vi "10 DAQ Config (PFI0) (2017).vi"(2 "Error In":errorcluster, 3 "rate":dbl=6000.0, 4 "number of samples":i32=240) -> (0 "Error Out":errorcluster, 1 "task out":refnum<k21>)   [LabVIEW 2017]
uses:
  <vilib>/DAQmx/create/channels.llb/DAQmx Create Channel (TEDS-AI-Voltage-Basic).vi
  <vilib>/DAQmx/create/channels.llb/DAQmx Create Channel (AI-Voltage-Basic).vi
  <vilib>/DAQmx/configure/timing.llb/DAQmx Timing (Sample Clock).vi
  <vilib>/DAQmx/configure/trigger.llb/DAQmx Trigger.vi
  <vilib>/DAQmx/configure/trigger.llb/DAQmx Start Trigger (Digital Edge).vi
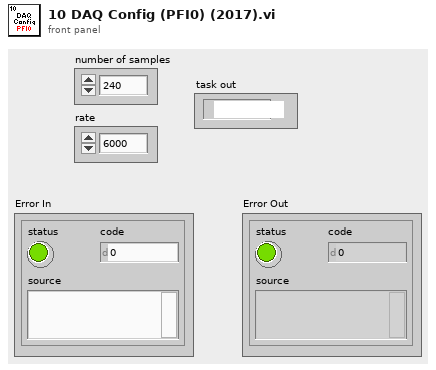
[diagram p1: front panel]
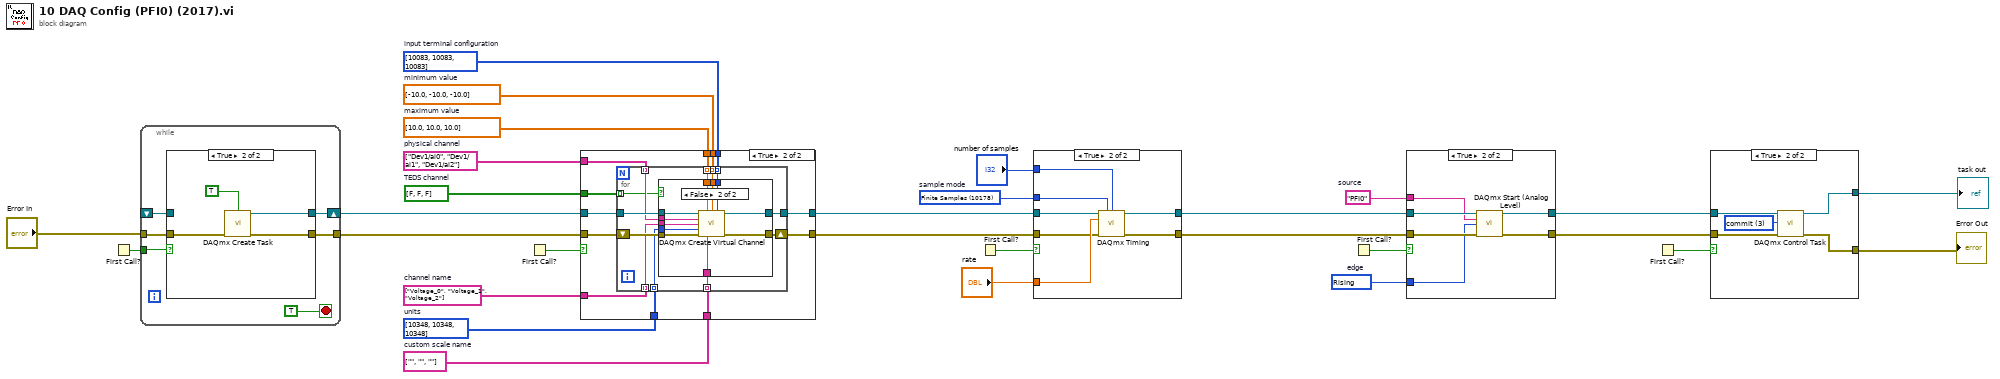
[diagram p0: block diagram]
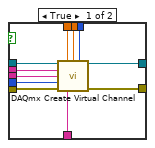
[diagram p6: hidden frame]
diagram:
  w26 = 10280 items=["Rising"=10280, "Falling"=10171]  # edge
  w25 = "PFI0"  # source
  w21 = 10178 items=["Finite Samples"=10178, "Continuous Samples"=10123, "Hardware Timed Single Point"=12522]  # sample mode
  w15 = bool[] [FALSE, FALSE, FALSE]  # TEDS channel
  w14 = string[] ["", "", ""]  # custom scale name
  w13 = i32[] [10348, 10348, 10348] items=["Volts"=10348, "From TEDS"=12516, "From Custom Scale"=10065]  # units
  w12 = string[] ["Voltage_0", "Voltage_1", "Voltage_2"]  # channel name
  w11 = string[] ["Dev1/ai0", "Dev1/ai1", "Dev1/ai2"]  # physical channel
  w10 = dbl[] [10.0, 10.0, 10.0]  # maximum value
  w9 = dbl[] [-10.0, -10.0, -10.0]  # minimum value
  w8 = i32[] [10083, 10083, 10083] items=["default"=-1, "RSE"=10083, "NRSE"=10078, "Differential"=10106, "Pseudodifferential"=12529]  # input terminal configuration
  n1 = First Call?() -> (First Call?: T/F=w3:bool)
  n2 = while {
    shift-right: [w34] -> w6
    shift-left: _ -> [w33]
    tunnel: w3 -> [w35]
    tunnel: [w32] -> w4
    tunnel: "Error In" -> [w31]
    stop <- TRUE stop-if-true
    n3 = case shown="True" w35 {
      tunnel: [w37 w41] -> w34
      tunnel: w33 -> [w37 _]
      tunnel: [w36 w40] -> w32
      tunnel: w31 -> [w36 w38]
      frame False {
      }
      frame True {
        n4 = call <vilib>:"DAQmx Create Task.vi"("auto cleanup"=TRUE, "error in"=w38) -> ("task out"=w41:refnum<k21>, "error out"=w40:errorcluster)  [unwired: 12 in]
      }
    }
  }
  n5 = First Call?() -> (First Call?: T/F=w5:bool)
  n6 = case shown="True" w5 {
    tunnel: [w43 w53] -> w17
    tunnel: w6 -> [w43 w55]
    tunnel: [w42 w52] -> w7
    tunnel: w4 -> [w42 w54]
    tunnel: w8 -> [_ w51]
    tunnel: w9 -> [_ w50]
    tunnel: w10 -> [_ w49]
    tunnel: w11 -> [_ w48]
    tunnel: w12 -> [_ w47]
    tunnel: w13 -> [_ w46]
    tunnel: w14 -> [_ w45]
    tunnel: w15 -> [_ w44]
    frame False {
    }
    frame True {
      n7 = for {
        tunnel: w55 -> [w67]
        tunnel: [w65] -> w53
        tunnel: w51 -> [w63] mode=indexing
        tunnel: w50 -> [w62] mode=indexing
        tunnel: w49 -> [w61] mode=indexing
        tunnel: w48 -> [w60] mode=indexing
        tunnel: w47 -> [w59] mode=indexing
        tunnel: w46 -> [w58] mode=indexing
        tunnel: w45 -> [w57] mode=indexing
        shift-right: [w64] -> w52
        shift-left: w54 -> [w66]
        tunnel: w44 -> [w56] mode=indexing
        n8 = case shown="False" w56 {
          tunnel: w67 -> [w78 w89]
          tunnel: w66 -> [w77 w88]
          tunnel: [w76 w87] -> w65
          tunnel: [w75 w86] -> w64
          tunnel: w63 -> [w74 w85]
          tunnel: w62 -> [w73 w84]
          tunnel: w61 -> [w72 w83]
          tunnel: w60 -> [w71 w82]
          tunnel: w59 -> [w70 w81]
          tunnel: w58 -> [w69 w80]
          tunnel: w57 -> [w68 w79]
          frame True {
            n9 = call-poly <vilib>:"DAQmx Create Virtual Channel.vi"("task in"=w78, "maximum value"=w72, "minimum value"=w73, "input terminal configuration"=w74, "physical channels"=w71, "name to assign"=w70, "units"=w69, "error in"=w77, "custom scale name"=w68) -> ("task out"=w76:refnum<k21>, "error out"=w75:errorcluster)  [unwired: 5 in]
          }
          frame False {
            n10 = call-poly <vilib>:"DAQmx Create Virtual Channel.vi"("task in"=w89, "maximum value"=w83, "minimum value"=w84, "input terminal configuration"=w85, "physical channels"=w82, "name to assign"=w81, "units"=w80, "error in"=w88, "custom scale name"=w79) -> ("task out"=w87:refnum<k21>, "error out"=w86:errorcluster)  [unwired: 5 in]
          }
        }
      }
    }
  }
  n11 = First Call?() -> (First Call?: T/F=w16:bool)
  n12 = case shown="True" w16 {
    tunnel: [w91 w93] -> w23
    tunnel: w17 -> [w91 w96]
    tunnel: [w90 w92] -> w18
    tunnel: w7 -> [w90 w94]
    tunnel: "number of samples" -> [_ w98]
    tunnel: w21 -> [_ w97]
    tunnel: "rate" -> [_ w95]
    frame False {
    }
    frame True {
      n13 = call-poly <vilib>:"DAQmx Timing.vi"("task/channels in"=w96, "sample mode"=w97, "samples per channel"=w98, "rate"=w95, "error in"=w94) -> ("task out"=w93:refnum<k21>, "error out"=w92:errorcluster)  [unwired: 9 in]
    }
  }
  n14 = First Call?() -> (First Call?: T/F=w22:bool)
  n15 = case shown="True" w22 {
    tunnel: [w100 w104] -> w28
    tunnel: w23 -> [w100 w106]
    tunnel: [w99 w103] -> w24
    tunnel: w18 -> [w99 w105]
    tunnel: w25 -> [_ w102]
    tunnel: w26 -> [_ w101]
    frame False {
    }
    frame True {
      n16 = call-poly "DAQmx Start (Analog Level).vi"("task/channels in"=w106, "source"=w102, "edge"=w101, "error in"=w105) -> ("task out"=w104:refnum<k21>, "error out"=w103:errorcluster)  [unwired: 10 in]
    }
  }
  n17 = First Call?() -> (First Call?: T/F=w27:bool)
  n18 = case shown="True" w27 {
    tunnel: [w108 w112] -> w29
    tunnel: w28 -> [w108 w113]
    tunnel: [w107 w110] -> w1
    tunnel: w24 -> [w107 w111]
    frame False {
    }
    frame True {
      w109 = 3 items=["verify"=2, "reserve"=4, "commit"=3, "unreserve"=5, "abort"=6] ("action")
      n19 = call <vilib>:"DAQmx Control Task.vi"("task/channels in"=w113, "action"=w109, "error in"=w111) -> ("task out"=w112:refnum<k21>, "error out"=w110:errorcluster)  [unwired: 11 in]
    }
  }
  "task out" <- w29
  "Error Out" <- w1
